vi "CurrentInstance.vi"() -> ()   [LabVIEW 2016, in "DronaTest.lvlib" / "test_Setup.lvlib"]
uses:
  test_Setup.lvlib
  <vilib>/addons/_JKI Toolkits/Caraya/classes/Assert/Assert Equal Value_Variant.vi
  <vilib>/addons/_JKI Toolkits/Caraya/classes/Test/Test.lvclass
  <vilib>/addons/_JKI Toolkits/Caraya/classes/Assert/Assert.lvclass
  main/Drona.lvlib
  main/apis/Setup/GetVI/GetVI.lvlib
panel:
  out "error out":errorcluster
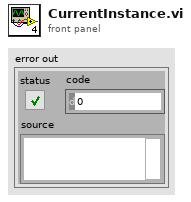
[diagram p1: front panel]
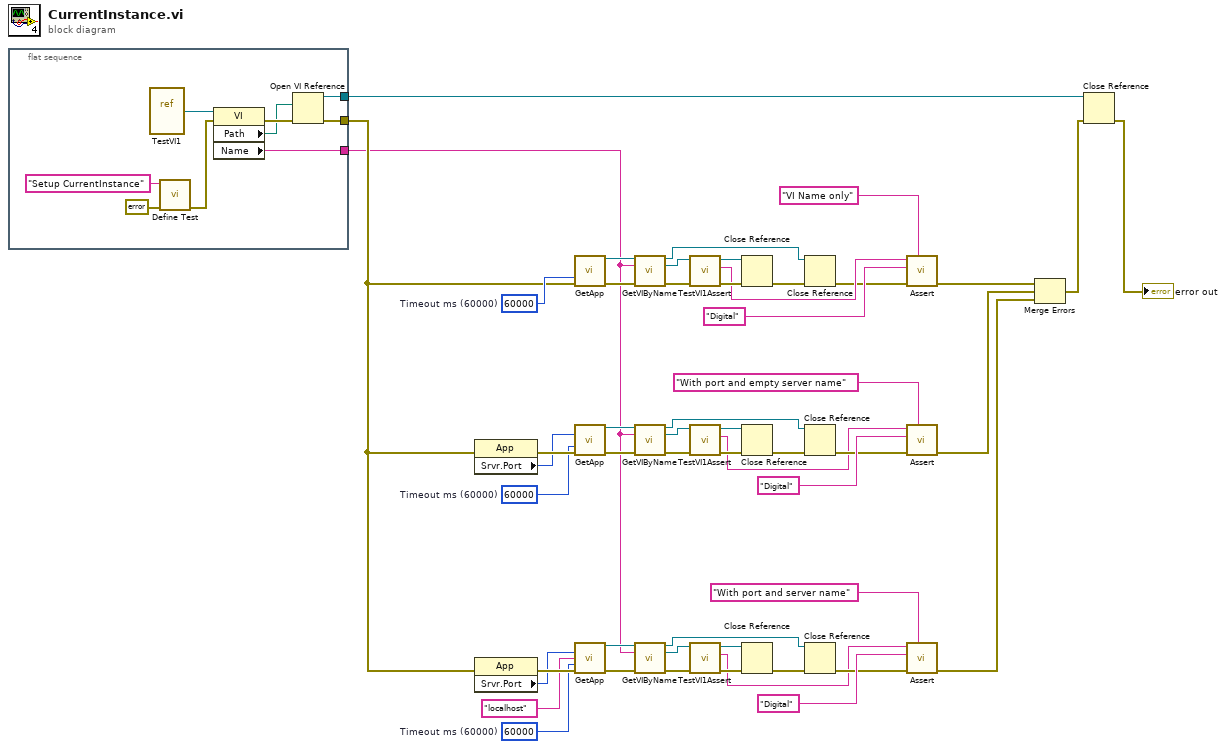
[diagram p0: block diagram]
diagram:
  w3 = 60000  # Timeout ms (60000)
  w16 = 60000  # Timeout ms (60000)
  w38 = 60000  # Timeout ms (60000)
  n1 = flat-sequence {
    tunnel: [w57] -> w33
    tunnel: [w56] -> w39
    tunnel: [w54] -> w1
    frame #0 {
      n2 = vi-ref "TestVI1.vi"() -> (w59:refnum<vi>)
      n3 = call <vilib>:"Define Test.vi"("error in (no error)"=errorcluster {"status"=FALSE, "code"=0, "source"=""}, "Label (VI Title)"="Setup CurrentInstance") -> ("error out"=w60:errorcluster)  [unwired: 9 in]
      n4 = property on="Property Node" class="VI"(reference=w59, error in=w60) -> (error out=w58:errorcluster, "Path"=w55:path, "Name"=w54:string)  [unwired: 1 out]
      n5 = Open VI Reference(vi path=w55, error in (no error)=w58) -> (vi reference=w56:refnum<vi>, error out=w57:errorcluster)  [unwired: 4 in]
    }
  }
  n6 = property on="Property Node" class="App"(error in=w33) -> (error out=w20:errorcluster, "Srvr.Port"=w17:u32)  [unwired: 1 in, 1 out]
  n7 = property on="Property Node" class="App"(error in=w33) -> (error out=w7:errorcluster, "Srvr.Port"=w5:u32)  [unwired: 1 in, 1 out]
  n8 = call "GetApp.vi"("Timeout ms (60000)"=w38, "error in (no error)"=w33) -> ("Application Ref"=w36:refnum<vi>, "error out"=w32:errorcluster)  [unwired: 12 in]
  n9 = call "GetApp.vi"("Port(0:Ignored)"=w17, "Timeout ms (60000)"=w16, "error in (no error)"=w20) -> ("Application Ref"=w24:refnum<vi>, "error out"=w27:errorcluster)  [unwired: 11 in]
  n10 = call "GetApp.vi"("Port(0:Ignored)"=w5, "Service Name (\"\":localhost)"="localhost" ("Service Name (\"\":localhost)"), "Timeout ms (60000)"=w3, "error in (no error)"=w7) -> ("Application Ref"=w12:refnum<vi>, "error out"=w9:errorcluster)  [unwired: 10 in]
  n11 = call "GetVIByName.vi"("Application Ref in"=w36, "VI Name"=w1, "error in (no error)"=w32) -> ("Application Ref out"=w35:refnum<vi>, "VI Reference"=w34:refnum<vi>, "error out"=w37:errorcluster)  [unwired: 10 in]
  n12 = call "GetVIByName.vi"("Application Ref in"=w24, "VI Name"=w1, "error in (no error)"=w27) -> ("Application Ref out"=w25:refnum<vi>, "VI Reference"=w26:refnum<vi>, "error out"=w23:errorcluster)  [unwired: 10 in]
  n13 = call "GetVIByName.vi"("Application Ref in"=w12, "VI Name"=w1, "error in (no error)"=w9) -> ("Application Ref out"=w11:refnum<vi>, "VI Reference"=w10:refnum<vi>, "error out"=w13:errorcluster)  [unwired: 10 in]
  n14 = call "TestVI1Assert.vi"("error in (no error)"=w37, "VI in"=w34) -> ("error out"=w50:errorcluster, "ClassName"=w48:string, "VI out"=w49:refnum<vi>)  [unwired: 7 in]
  n15 = call "TestVI1Assert.vi"("error in (no error)"=w23, "VI in"=w26) -> ("error out"=w21:errorcluster, "ClassName"=w18:string, "VI out"=w22:refnum<vi>)  [unwired: 7 in]
  n16 = call "TestVI1Assert.vi"("error in (no error)"=w13, "VI in"=w10) -> ("error out"=w15:errorcluster, "ClassName"=w2:string, "VI out"=w14:refnum<vi>)  [unwired: 7 in]
  n17 = Close Reference(reference=w49, error in (no error)=w50) -> (error out=w30:errorcluster)
  n18 = Close Reference(reference=w22, error in (no error)=w21) -> (error out=w28:errorcluster)
  n19 = Close Reference(reference=w14, error in (no error)=w15) -> (error out=w8:errorcluster)
  n20 = Close Reference(reference=w35, error in (no error)=w30) -> (error out=w29:errorcluster)
  n21 = Close Reference(reference=w25, error in (no error)=w28) -> (error out=w19:errorcluster)
  n22 = Close Reference(reference=w11, error in (no error)=w8) -> (error out=w6:errorcluster)
  n23 = call-poly <vilib>:"Assert.vi"("Label"="VI Name only" ("Label (VI Title)"), "error in (no error)"=w29, "Y"="Digital" ("Class Name"), "X"=w48) -> ("error out"=w51:errorcluster)  [unwired: 7 in]
  n24 = call-poly <vilib>:"Assert.vi"("Label"="With port and empty server name" ("Label (VI Title)"), "error in (no error)"=w19, "Y"="Digital" ("Class Name"), "X"=w18) -> ("error out"=w44:errorcluster)  [unwired: 7 in]
  n25 = call-poly <vilib>:"Assert.vi"("Label"="With port and server name" ("Label (VI Title)"), "error in (no error)"=w6, "Y"="Digital" ("Class Name"), "X"=w2) -> ("error out"=w41:errorcluster)  [unwired: 7 in]
  n26 = Merge Errors(w51, w44, w41) -> (w31:errorcluster)
  n27 = Close Reference(reference=w39, error in (no error)=w31) -> (error out=→"error out":errorcluster)
